vi "Get TestSuite Test Paths.vi"(8 "error in (no error)":errorcluster, 11 "Test Project":path) -> (0 "error out":errorcluster, 2 "Test Paths":path[](array[path]))   [LabVIEW 2011, in "GraphicalTestRunner.lvlib"]
uses:
  GraphicalTestRunner.lvlib
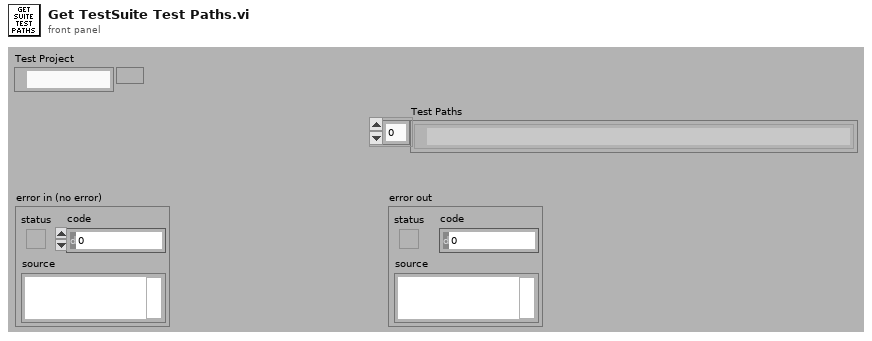
[diagram p1: front panel]
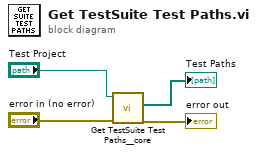
[diagram p0: block diagram]
diagram:
  n1 = call "Get TestSuite Test Paths__core.vi"("error in (no error)"="error in (no error)", "Test Project"="Test Project") -> ("error out"=→"error out":errorcluster, "Test Paths"=→"Test Paths":path[])  [unwired: 8 in]
